vi "5302GetSensitivity.vi"(8 "error in (no error)":errorcluster, 11 "VISA Resource Name":refnum<visa-resource-name>) -> (0 "error out":errorcluster, 1 "data string":string, 2 "Sevsitivity":dbl format="%.4e", 3 "VISA Resource Name Out":refnum<visa-resource-name>)   [LabVIEW 2015]
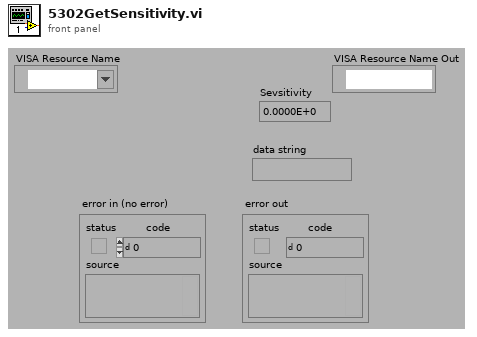
[diagram p1: front panel]
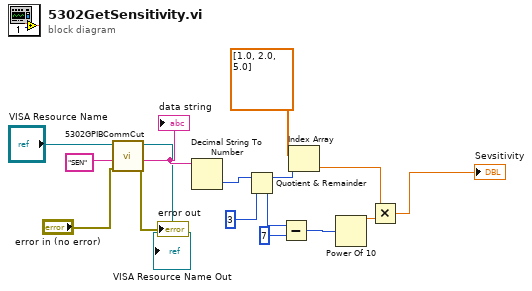
[diagram p0: block diagram]
diagram:
  n1 = call "5302GPIBCommCut.vi"("error in (no error)"="error in (no error)", "data string in"="SEN" ("data string"), "VISA Resource Name"="VISA Resource Name") -> ("error out"=→"error out":errorcluster, "data string out"=w10:string, "VISA Resource Name Out"=→"VISA Resource Name Out":refnum<visa-resource-name>)  [unwired: 2 in, 4 out]
  "data string" <- w10
  n2 = Decimal String To Number(string=w10) -> (number=w9:i32)  [unwired: 1 in, 2 out]
  n3 = Quotient & Remainder(x=w9, y=3) -> (x-y*floor(x/y)=w5:i32, floor(x/y)=w7:i32)
  n4 = Subtract(x=w7, y=7) -> (x-y=w8:i32)
  n5 = Index Array(array=dbl[] [1.0, 2.0, 5.0] ("Input Array"), index=w5) -> (element=w3:dbl)
  n6 = Power Of 10(x=w8) -> (10^x=w12:dbl)
  n7 = Multiply(x=w3, y=w12) -> (x*y=→"Sevsitivity":dbl)
